vi "RemoteControl.TestLauncher.ConnectionMonitor.vi"(6 "Commands":string="Command1\nCommand2\nCommand3\nCMD WITH SPACE\nACK\nHELP", 8 "error in (no error)":errorcluster, 9 "port":u16=6341, 10 "address":string="*", 11 "RemoteControl in":refnum<class "RemoteControl.lvclass">) -> (0 "error out":errorcluster)   [LabVIEW 2019, in "RemoteControl.lvlib" / "RemoteControl.lvclass"]
uses:
  RemoteControl.lvclass
  <vilib>/JKI/JKI SMO/SMO/Typedefs/SMOState --Enum.ctl
  C:/Program Files/National Instruments/LabVIEW 2019/vi.lib/JKI/JKI SMO/SMO/SMO.lvclass
  Typedefs/RC Process Type--Enum.ctl
  <userlib>/LevyLab/Debug/Attribute.Debug/DebugBehavior.ctl
  RemoteControl.lvclass/RemoteControl.ctl
  <vilib>/JKI/JKI SMO/SMO/SMO.lvclass/SMO.ctl
  <vilib>/JKI/JKI SMO/SMO/Private/ReftoDVR--SMO.vi
  <userlib>/LevyLab/Debug/Debug.lvlib
  <userlib>/LevyLab/Debug/Attribute.Debug/Attribute.Debug.lvclass
  <vilib>/JKI/JKI SMO/SMO/SMO.lvclass
panel:
  out "message (response)":string="Command: ACK\nID: AD5B483F-0643-4E65-A894-29EB599D2C28\nData:\n\tCommand: ACK\n\tTime: 10:15:51 PM\n\tGUID: A1E7D8EE-9379-462A-9A6B-E1EB887A3889"
  out "message (request)":string="Command: ACK\nID: AD5B483F-0643-4E65-A894-29EB599D2C28\nData:\n\t25330.725758"
  in  "delay response":bool
  in  "RC Process Type":T1=enum."Server"
  in  "Debug Mode":bool=TRUE
  in  "Check Timing Mode":bool
  out "processed":i32=4050
  out "SMO State":T2=enum."Stopped"
  in  "Stop":bool
  # "Remote Control Launcher"
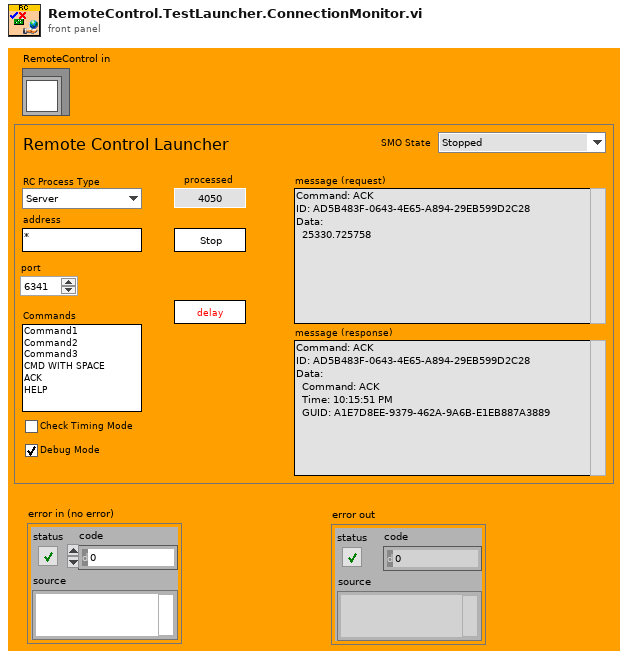
[diagram p1: front panel]
types:
  T1 = typedef "RemoteControl.lvlib/RemoteControl.lvclass/RC Process Type--Enum.ctl" = enum16{"Listener", "Server", "Client"}
  T2 = typedef "SMO.lvclass/SMOState --Enum.ctl" = enum16{"unknown", "Created", "Started", "Stopped"}
  T3 = typedef "Debug.lvlib/Attribute.Debug.lvclass/DebugBehavior.ctl" = enum16{"Normal", "Debug"}
  T4 = typedef "SMO.lvclass/Public Events.ctl" = cluster{"Error":refnum<user-event>, "State":refnum<user-event>, "Reserve State":refnum<user-event>}
  T5 = typedef "RemoteControl.lvlib/RemoteControl.lvclass/PublicEvents--Cluster.ctl" = cluster{"SendMessageFromProcess":refnum<user-event>}
  T6 = typedef "RemoteControl.lvlib/RemoteControl.lvclass/Message--Cluster.ctl" = cluster{"Command":string, "Data":variant, "ID":string, "error":errorcluster}
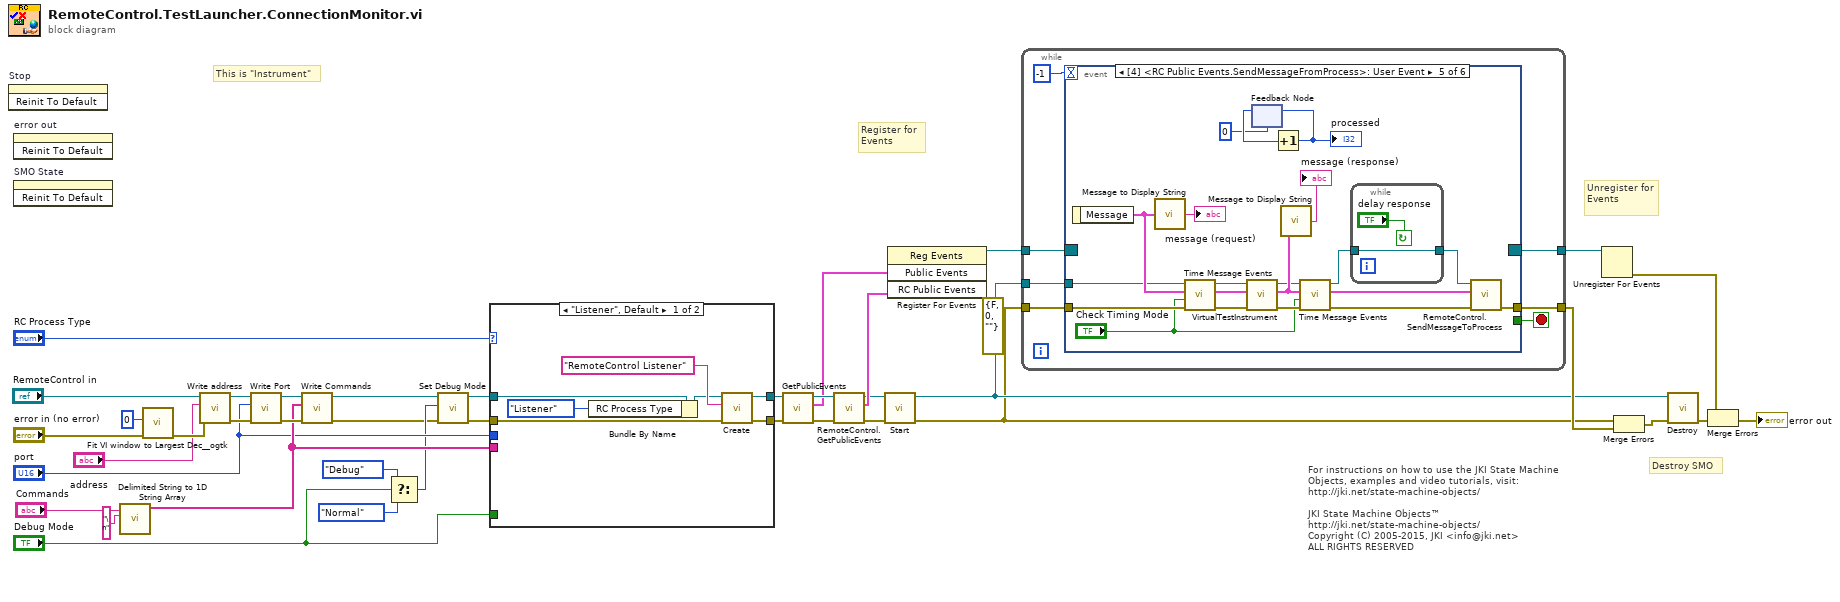
[diagram p0: block diagram]
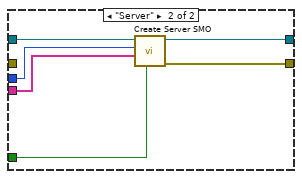
[diagram p2: hidden frame]
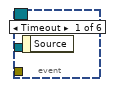
[diagram p3: hidden frame]
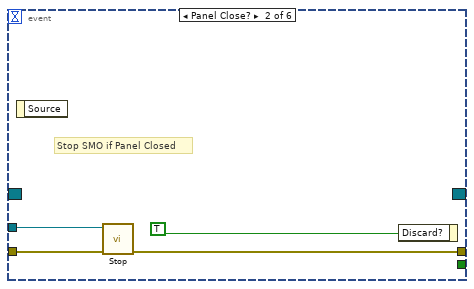
[diagram p4: hidden frame]
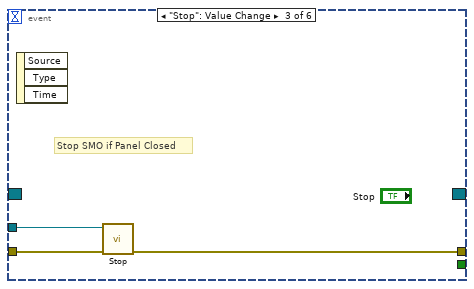
[diagram p5: hidden frame]
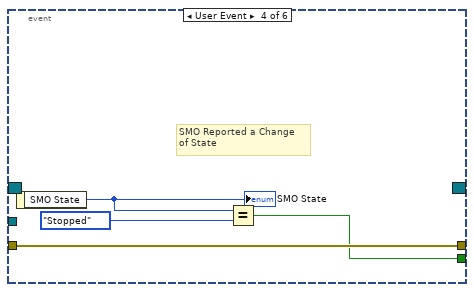
[diagram p6: hidden frame]
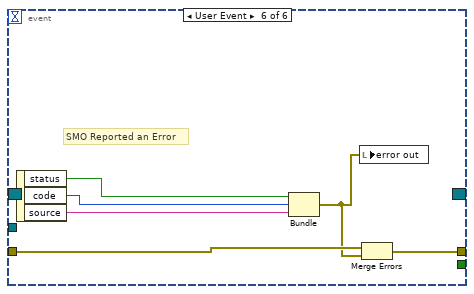
[diagram p7: hidden frame]
diagram:
  (unwired) errorcluster {"status"=FALSE, "code"=0, "source"=""} ("error out")
  # "Register for Events"
  # "This is \"Instrument\""
  # "For instructions on how to use the JKI State Machine Objects, examples and video tutorials, visit:\nhttp://jki.net/state-machine-objects/\n\nJKI State Machine Objects™\nhttp://jki.net/state-machine-objects/\nCopyright (C) 2005-2015, JKI <info@jki.net>\nALL RIGHTS RESERVED"
  # "Destroy SMO"
  # "Unregister for Events"
  n1 = invoke on="Stop" class="Bool" method="Reinit To Default"() -> ()  [unwired: 3 in, 3 out]
  n2 = invoke on="error out" class="Clust (strict)" method="Reinit To Default"() -> ()  [unwired: 3 in, 3 out]
  n3 = invoke on="SMO State" class="Enum (strict)" method="Reinit To Default"() -> ()  [unwired: 3 in, 3 out]
  n4 = call <vilib>:"Delimited String to 1D String Array.vi"("delimiter"="\n", "delimited string"="Commands") -> ("string array"=w11:string[])  [unwired: 9 in]
  n5 = call <userlib>:"Fit VI window to Largest Dec__ogtk.vi"("error in (no error)"="error in (no error)", "border spacing (2 px)"=0) -> ("error out"=w14:errorcluster)  [unwired: 4 in, 1 out]
  n6 = call-dynamic "Write address.vi"("error in (no error)"=w14, "address"="address", "RemoteControl in"="RemoteControl in") -> ("error out"=w27:errorcluster, "RemoteControl out"=w28:refnum<class "RemoteControl.lvclass">)  [unwired: 7 in]
  n7 = call-dynamic "Write Port.vi"("error in (no error)"=w27, "Port"="port", "RemoteControl in"=w28) -> ("error out"=w25:errorcluster, "RemoteControl out"=w26:refnum<class "RemoteControl.lvclass">)  [unwired: 7 in]
  n8 = call-dynamic "Write Commands.vi"("error in (no error)"=w25, "Commands"=w11, "RemoteControl in"=w26) -> ("error out"=w4:errorcluster, "RemoteControl out"=w5:refnum<class "RemoteControl.lvclass">)  [unwired: 7 in]
  n9 = Select(t=DebugBehavior."Debug" ("Behavior"), s="Debug Mode", f=DebugBehavior."Normal" ("Behavior")) -> (s? t:f=w7:T3)
  n10 = call <userlib>:"Set Debug Mode.vi"("error in (no error)"=w4, "Behavior"=w7, "SMO"=w5) -> ("error out"=w3:errorcluster, "SMO out"=w6:refnum<class "RemoteControl.lvclass">)  [unwired: 7 in]
  n11 = case shown="\"Listener\", Default" "RC Process Type" {
    tunnel: [w43 w52] -> w24
    tunnel: [w44 w51] -> w23
    tunnel: w6 -> [w42 w48]
    tunnel: w3 -> [w41 _]
    tunnel: "port" -> [_ w47]
    tunnel: w11 -> [_ w50]
    tunnel: "Debug Mode" -> [_ w49]
    frame "Listener", Default {
      n12 = Bundle By Name(cluster=w42, "RC Process Type"=RC_Process_Type--Enum."Listener") -> (w40:refnum<class "RemoteControl.lvclass">)
      n13 = call <vilib>:"Create.vi"("error in (no error)"=w41, "Subsystem Name (optional)"="RemoteControl Listener" ("format string"), "SMO"=w40) -> ("error out"=w44:errorcluster, "SMO out"=w43:refnum<class "RemoteControl.lvclass">)  [unwired: 6 in, 1 out]
    }
    frame "Server" {
      n14 = call "Create Server SMO.vi"("Debug Mode?"=w49, "Commands"=w50, "Port"=w47, "RemoteControl in"=w48) -> ("error out"=w51:errorcluster, "RemoteControl out"=w52:refnum<class "RemoteControl.lvclass">)  [unwired: 6 in]
    }
  }
  n15 = call <vilib>:"GetPublicEvents.vi"("error in (no error)"=w23, "SMO"=w24) -> ("error out"=w33:errorcluster, "Public Events"=w32:T4, "SMO out"=w34:refnum<class "RemoteControl.lvclass">)  [unwired: 7 in]
  n16 = call "RemoteControl.GetPublicEvents.vi"("error in (no error)"=w33, "RemoteControl"=w34) -> ("error out"=w22:errorcluster, "RC Public Events"=w30:T5, "RemoteControl out"=w21:refnum<class "RemoteControl.lvclass">)  [unwired: 7 in]
  n17 = call <vilib>:"Start.vi"("error in (no error)"=w22, "SMO"=w21) -> ("error out"=w19:errorcluster, "SMO out"=w20:refnum<class "RemoteControl.lvclass">)  [unwired: 8 in]
  n18 = register-events(w32, w30) -> (reference out=w31:refnum<event-registration>)  [unwired: 2 in, 1 out]
  n19 = while {
    tunnel: w31 -> [w56]
    tunnel: [w55] -> w39
    tunnel: w20 -> [w54]
    tunnel: w19 -> [w57]
    tunnel: [w58] -> w38
    stop <- w59 stop-if-true
    n20 = event shown="[4] <RC Public Events.SendMessageFromProcess>: User Event" {
      selector: w56 -> [_ _ _ _ _ _]
      dyn-events: [_ _ _ _ _ _] -> w55
      timeout: -1 -> [_ _ _ _ _ _]
      tunnel: [_ _ _ w67 _ _] -> w59
      tunnel: w54 -> [_ w63 w66 _ w75 _]
      tunnel: [_ w62 w65 w70 _ w96] -> w58
      tunnel: w57 -> [_ w61 w64 w70 w86 w94]
      tunnel: [_ _ _ _ w90 _] -> _
      event Timeout {
        n21 = event-data() -> ()  [unwired: 1 in, 1 out]
      }
      event Panel Close? {
        # "Stop SMO if Panel Closed"
        n22 = event-data() -> ()  [unwired: 1 in, 1 out]
        n23 = call <vilib>:"Stop.vi"("error in (no error)"=w61, "SMO"=w63) -> ("error out"=w62:errorcluster)  [unwired: 8 in, 1 out]
        n24 = event-data("Discard?"=TRUE ("OK")) -> ()  [unwired: 1 in, 1 out]
      }
      event "Stop": Value Change {
        # "Stop SMO if Panel Closed"
        n25 = event-data() -> ()  [unwired: 1 in, 3 out]
        n26 = call <vilib>:"Stop.vi"("error in (no error)"=w64, "SMO"=w66) -> ("error out"=w65:errorcluster)  [unwired: 8 in, 1 out]
      }
      event User Event {
        # "SMO Reported a Change\nof State"
        n27 = event-data() -> ("SMO State"=w69:T2)  [unwired: 1 in]
        "SMO State" <- w69
        n28 = Equal?(x=w69, y=SMOState_--Enum."Stopped") -> (x = y?=w67:bool)
      }
      event User Event {
        n29 = event-data() -> ("Message"=w80:T6)  [unwired: 1 in]
        n30 = call "Message to Display String.vi"("Message"=w80) -> ("message string"=→"message (request)":string)
        n31 = call "Time Message Events.vi"("error in (no error)"=w86, "Debug Mode"="Check Timing Mode", "Message in"=w80, "RemoteControl"=w75) -> ("error out"=w85:errorcluster, "Message out"=w79:T6, "RemoteControl out"=w74:refnum<class "RemoteControl.lvclass">)  [unwired: 4 in, 1 out]
        n32 = call "VirtualTestInstrument.vi"("error in (no error)"=w85, "Message"=w79, "RemoteControl"=w74) -> ("error out"=w83:errorcluster, "processed Message"=w76:T6, "RemoteControl"=w73:refnum<class "RemoteControl.lvclass">)  [unwired: 6 in]
        n33 = feedback #1(0) -> (w88:i32)
        n34 = Increment(x=w88) -> (x+1=w89:i32)
        "processed" <- w89
        n35 = feedback-in #1(w89) -> ()
        n36 = call "Message to Display String.vi"("Message"=w76) -> ("message string"=→"message (response)":string)
        n37 = call "Time Message Events.vi"("error in (no error)"=w83, "Debug Mode"="Check Timing Mode", "Message in"=w76, "RemoteControl"=w73) -> ("error out"=w84:errorcluster, "Message out"=w78:T6, "RemoteControl out"=w72:refnum<class "RemoteControl.lvclass">)  [unwired: 4 in, 1 out]
        n38 = while {
          tunnel: [w91] -> w82
          tunnel: w72 -> [w91]
          stop <- "delay response" continue-if-true
        }
        n39 = call "RemoteControl.SendMessageToProcess.vi"("error in (no error)"=w84, "Message"=w78, "RemoteControl"=w82) -> ("error out"=w90:errorcluster)  [unwired: 7 in, 1 out]
      }
      event User Event {
        # "SMO Reported an Error"
        n40 = event-data() -> ("status"=w95:bool, "code"=w98:i32, "source"=w97:string)  [unwired: 1 in]
        n41 = Bundle("status"=w95, "code"=w98, "source"=w97) -> (w93:errorcluster)  [unwired: 1 in]
        n42 = local write "error out"(w93) -> ()
        n43 = Merge Errors(w94, w93) -> (w96:errorcluster)
      }
    }
  }
  n44 = Unregister For Events(event registration refnum=w39) -> (error out=w37:errorcluster)  [unwired: 1 in]
  n45 = Merge Errors(w19, w38) -> (w29:errorcluster)
  n46 = call <vilib>:"Destroy.vi"("error in (no error)"=w29, "SMO"=w20) -> ("error out"=w35:errorcluster)  [unwired: 9 in]
  n47 = Merge Errors(w37, w35) -> (→"error out":errorcluster)
